vi "Day 8.2 - .vi"(11 "input":i32[][](array[numeric])) -> (3 "output":u64)   [LabVIEW 2021]
panel:
  out "Scores":i32[][](array[numeric])
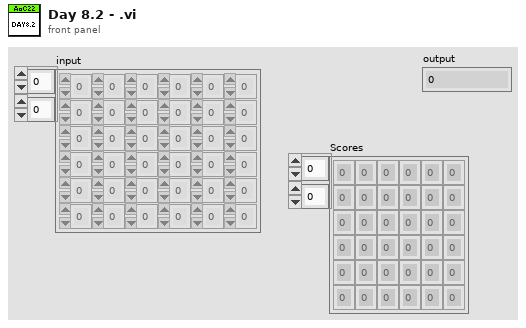
[diagram p1: front panel]
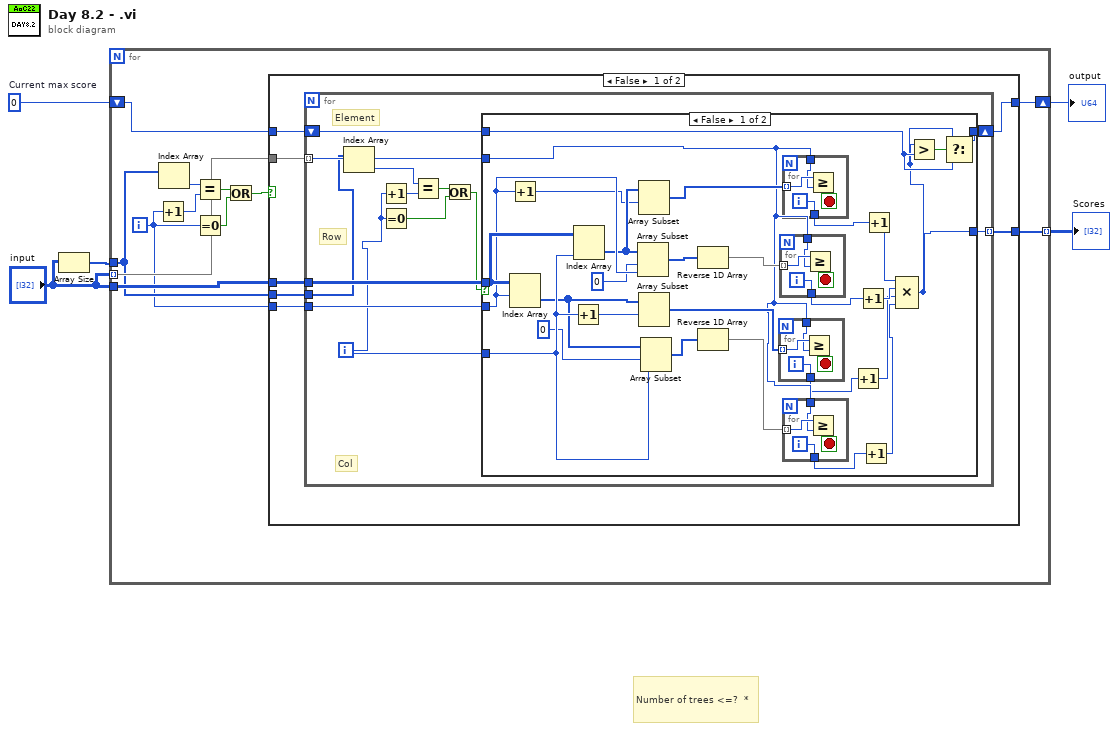
[diagram p0: block diagram]
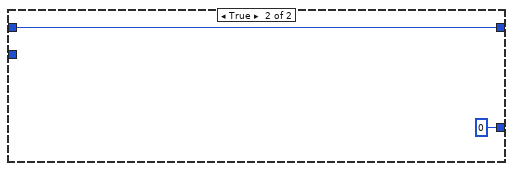
[diagram p2: hidden frame]
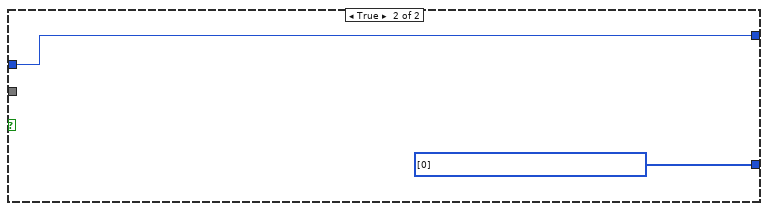
[diagram p3: hidden frame]
diagram:
  w3 = u64 0  # Current max score
  # "Number of trees <=?  *"
  n1 = Array Size(array="input") -> (size(s)=w5:i32[])
  n2 = for {
    tunnel: "input" -> [w17] mode=indexing
    tunnel: "input" -> [w16]
    tunnel: w5 -> [w8]
    shift-right: [w14] -> w2
    shift-left: w3 -> [w15]
    tunnel: [w13] -> w1 mode=indexing
    i -> [w7]
    n3 = Increment(x=w7) -> (x+1=w11:i32)
    n4 = Index Array(array=w8) -> (element=w12:i32)  [unwired: 1 in]
    n5 = Equal?(x=w12, y=w11) -> (x = y?=w10:bool)
    n6 = Equal To 0?(x=w7) -> (x = 0?=w9:bool)
    n7 = Or(x=w10, y=w9) -> (x .or. y?=w6:bool)
    n8 = case shown="False" w6 {
      tunnel: w17 -> [w24 _]
      tunnel: w16 -> [w23 _]
      tunnel: w15 -> [w22 w85]
      tunnel: [w21 w85] -> w14
      tunnel: [w20 i32[] [0]] -> w13
      tunnel: w8 -> [w19 _]
      tunnel: w7 -> [w18 _]
      frame False {
        n9 = for {
          tunnel: w24 -> [w35] mode=indexing
          tunnel: w23 -> [w37]
          tunnel: w19 -> [w27]
          tunnel: w18 -> [w36]
          shift-right: [w33] -> w21
          shift-left: w22 -> [w34]
          tunnel: [w32] -> w20 mode=indexing
          i -> [w26]
          # "Col"
          # "Row"
          # "Element"
          n10 = Index Array(array=w27) -> (element=w28:i32)  [unwired: 1 in]
          n11 = Increment(x=w26) -> (x+1=w29:i32)
          n12 = Equal To 0?(x=w26) -> (x = 0?=w31:bool)
          n13 = Equal?(x=w28, y=w29) -> (x = y?=w30:bool)
          n14 = Or(x=w30, y=w31) -> (x .or. y?=w25:bool)
          n15 = case shown="False" w25 {
            tunnel: w37 -> [w65 _]
            tunnel: w26 -> [w64 _]
            tunnel: w36 -> [w63 _]
            tunnel: w35 -> [w50 _]
            tunnel: w34 -> [w40 w82]
            tunnel: [w39 w82] -> w33
            tunnel: [w38 0] -> w32
            frame False {
              n16 = Increment(x=w63) -> (x+1=w58:i32)
              n17 = Index Array(array=w65, index (row)=w63) -> (element=w59:i32[])  [unwired: 1 in]
              n18 = Increment(x=w64) -> (x+1=w57:i32)
              n19 = Index Array(array=w65, index (col)=w64) -> (element=w60:i32[])  [unwired: 1 in]
              n20 = Array Subset(array=w60, index=0, length=w63) -> (w56:i32[])
              n21 = Array Subset(array=w60, index=w58) -> (w54:i32[])  [unwired: 1 in]
              n22 = Array Subset(array=w59, index=w57) -> (w52:i32[])  [unwired: 1 in]
              n23 = Array Subset(array=w59, index=0, length=w64) -> (w55:i32[])
              n24 = Reverse 1D Array(array=w56) -> (reversed array=w53:i32[])
              n25 = Reverse 1D Array(array=w55) -> (reversed array=w51:i32[])
              n26 = for {
                tunnel: w52 -> [w73] mode=indexing
                tunnel: w50 -> [w72]
                tunnel: [w70] -> w47
                i -> [w70]
                stop <- w71 stop-if-true
                n27 = Greater Or Equal?(x=w73, y=w72) -> (x >= y?=w71:bool)
              }
              n28 = for {
                tunnel: w53 -> [w77] mode=indexing
                tunnel: w50 -> [w76]
                tunnel: [w74] -> w48
                i -> [w74]
                stop <- w75 stop-if-true
                n29 = Greater Or Equal?(x=w77, y=w76) -> (x >= y?=w75:bool)
              }
              n30 = for {
                tunnel: w54 -> [w81] mode=indexing
                tunnel: w50 -> [w80]
                tunnel: [w78] -> w49
                i -> [w78]
                stop <- w79 stop-if-true
                n31 = Greater Or Equal?(x=w81, y=w80) -> (x >= y?=w79:bool)
              }
              n32 = for {
                tunnel: w51 -> [w69] mode=indexing
                tunnel: w50 -> [w68]
                tunnel: [w66] -> w46
                i -> [w66]
                stop <- w67 stop-if-true
                n33 = Greater Or Equal?(x=w69, y=w68) -> (x >= y?=w67:bool)
              }
              n34 = Increment(x=w47) -> (x+1=w43:i32)
              n35 = Increment(x=w48) -> (x+1=w44:i32)
              n36 = Increment(x=w46) -> (x+1=w42:i32)
              n37 = Increment(x=w49) -> (x+1=w45:i32)
              n38 = Compound Arithmetic op=MULTIPLY(w45, w44, w43, w42) -> (w38:i32)
              n39 = Greater?(x=w38, y=w40) -> (0:w41:bool)
              n40 = Select(t=w38, s=w41, f=w40) -> (s? t:f=w39:u64)
            }
            frame True {
            }
          }
        }
      }
      frame True {
      }
    }
  }
  "output" <- w2
  "Scores" <- w1
